vi "Bars.vi"() -> ()   [LabVIEW 2012]
uses:
  <vilib>/Platform/TimedLoop/XDataNode/timing_clust.ctl
  <vilib>/Platform/TimedLoop/XDataNode/nitl_modes.ctl
  <vilib>/Platform/TimedLoop/XDataNode/wakeup.ctl
  <vilib>/platform/TimedLoop/XDataNode/XDataNode.xnode
  <vilib>/Platform/TimedLoop/XDataNode/XDNodeRunTimeDep.lvlib
panel:
  in  "Tabs":enum32{"Display", "Setup"}(tab)
  out "Picture":picture
  in  "Bar width":dbl=2.0
  in  "Bar speed":dbl=10.0
  in  "Monitor scale":dbl=40.0
  in  "Amplitude":dbl
  in  "Frequency":dbl
  in  "Color":u32(colorbox)
  in  "Stop":bool
  # "cm"
  # "cm/sec"
  # "pix/cm"
  # "cm/sec"
  # "Hz"
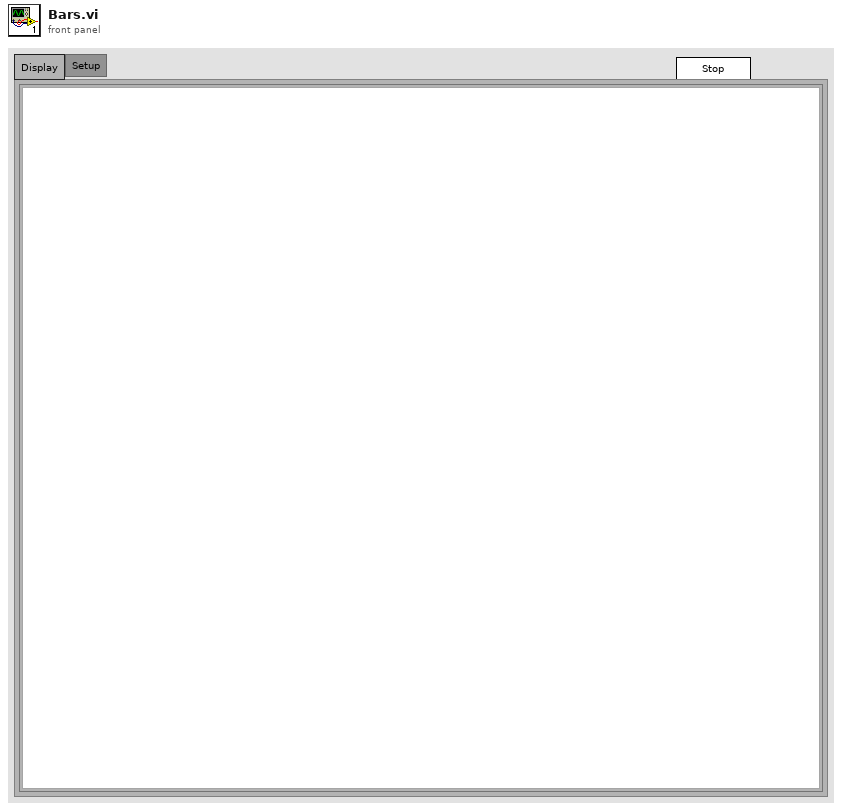
[diagram p1: front panel]
types:
  T1 = typedef "LVBoundsTypeDef.ctl" = cluster{"Width":u32, "Height":u32}
  T2 = typedef "XDNodeRunTimeDep.lvlib/timing_clust.ctl" = cluster{"Expected End [f-1]":u64, "Actual End [f-1]":u64, "Finished Late? [f-1]":bool, "Expected End [i-1]":u64, "Actual End [i-1]":u64, "Finished Late? [i-1]":bool, "Expected Start [i]":u64, "Actual Start [i]":u64, "Expected Start [f]":u64, "Actual Start [f]":u64, "Source Name":string, "Structure Name":string, "Period":i64, "Deadline":i64, "Offset":i64, "Start":i64, "Priority":i32, "Timeout":i32, "Mode":T3, "Wakeup Reason":T4, "Error":errorcluster, "Source Type":string, "Secondary Source Type":string, "Global End Time":u64, "Global Start Time":u64, "Frame Duration":u64, "Iteration Duration":u64, "Assigned CPU":i32, "I/O Scan Engine Mode":u32}
  T3 = typedef "XDNodeRunTimeDep.lvlib/nitl_modes.ctl" = enum32{"No Change", "Process missed periods, maintain original phase", "Discard missed periods, maintain original phase", "Process missed periods, ignore original phase", "Discard missed periods, ignore original phase"}
  T4 = typedef "XDNodeRunTimeDep.lvlib/wakeup.ctl" = enum32{"Normal", "Aborted", "Asynchronous wakeup", "Timing source error", "Timed loop error", "Timeout"}
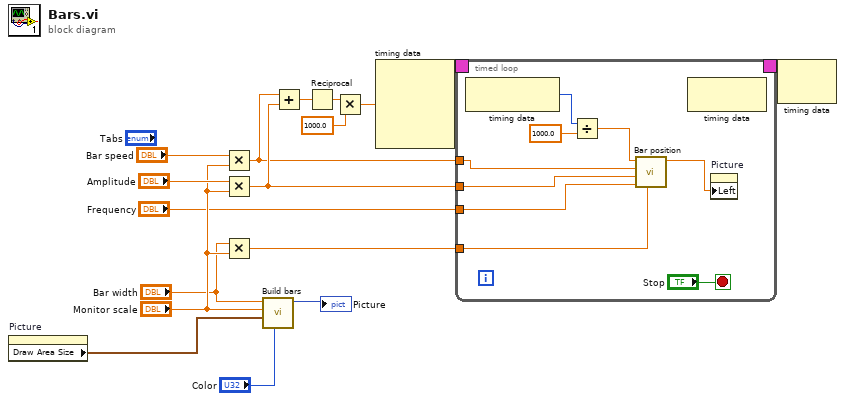
[diagram p0: block diagram]
diagram:
  n1 = property on="Picture" class="Pict"() -> ("Draw Area Size"=w17:T1)  [unwired: 2 in, 2 out]
  n2 = Multiply(x="Bar speed", y="Monitor scale") -> (x*y=w2:dbl)
  n3 = Multiply(x="Amplitude", y="Monitor scale") -> (x*y=w3:dbl)
  n4 = Multiply(x="Bar width", y="Monitor scale") -> (x*y=w9:dbl)
  n5 = call "Build bars.vi"("color(black)"="Color", "Draw Area Size"=w17, "Monitor scale"="Monitor scale", "Bar width"="Bar width") -> ("bars"=→"Picture":picture)  [unwired: 7 in]
  n6 = Add(x=w2, y=w3) -> (x+y=w4:dbl)
  n7 = Reciprocal(x=w4) -> (1/x=w10:dbl)
  n8 = Multiply(x=w10, y=1000.0) -> (x*y=w11:dbl)
  n9 = node-c288(w11) -> (w14:T2)  [unwired: 3 in]
  n10 = timed-loop {
    timing: w14 -> [_]
    timing-out: [_] -> w13
    tunnel: w2 -> [w22]
    tunnel: w9 -> [w20]
    tunnel: w3 -> [w19]
    tunnel: "Frequency" -> [w18]
    stop <- "Stop" stop-if-true
    n11 = node-c288() -> (w25:i64)  [unwired: 1 in]
    n12 = Divide(x=w25, y=1000.0) -> (x/y=w23:dbl)
    n13 = call "Bar position.vi"("bar width (pix)"=w20, "frequency (Hz)"=w18, "amplitude (pix/s)"=w19, "speed (pix/s)"=w22, "time (s)"=w23) -> ("position out"=w21:dbl)  [unwired: 6 in]
    n14 = node-c288() -> ()  [unwired: 1 in, 1 out]
    n15 = property on="Picture" class="Pict"("Left"=w21) -> ()  [unwired: 2 in, 2 out]
  }
  n16 = node-c288(w13) -> ()  [unwired: 1 out]
